vi "Calculate Load Current Array.vi"(8 "error in":errorcluster, 11 "measurement configuration":T1={"Mode of operation"=enum."Perform measurement", "DUT setup time"=1.0, "Source delay"=0.005, "Aperture time"=0.005, "Nominal output voltage"=3.3, "Source pin name"="", "Source sense"=1009, "Source current limit"=25.0, "Source maximum power"=300.0, "Source start voltage"=5.0, "Source stop voltage"=20.0, "Source voltage sweep points"=10, "Use Source voltage array"=FALSE, "Source voltage array"=[], "Load pin name"="", "Load sense"=1009, "Load voltage limit range"=6.0, "Load sweep type"="Logarithmic", "Load start current"=0.1, "Load stop current"=24.0, "Load current sweep points/points per decade"=10, "Use Load current array"=FALSE, "Load current array"=[], "Pin Names for Scope"=[], "vertical range"=[], "vertical offset"=[], "probe attenuation"=[], "vertical coupling"=[], "channel enabled"=[], "input impedance"=[], "max input frequency"=[], "min sample rate"=[], "reference position"=[], "min record length"=[], "enforce realtime"=[]} {"input impedance" items=["1 mega ohm"=0, "50 ohms"=2]; "vertical coupling" items=["AC", "DC", "Ground"]; "Load sense" items=["Local"=1008, "Remote"=1009]; "Source sense" items=["Local"=1008, "Remote"=1009]}) -> (0 "error out":errorcluster, 2 "Load current array size":i32, 3 "Load current array":dbl[](array[numeric]))   [LabVIEW 2021, in "Efficiency And Load Regulation with Pin Map.lvlib"]
uses:
  Efficiency And Load Regulation with Pin Map.lvlib
  Measurement Configuration.ctl
  <instrlib>/niScope/Controls/niScope vertical coupling.ctl
  common/PMIC Common.lvlib
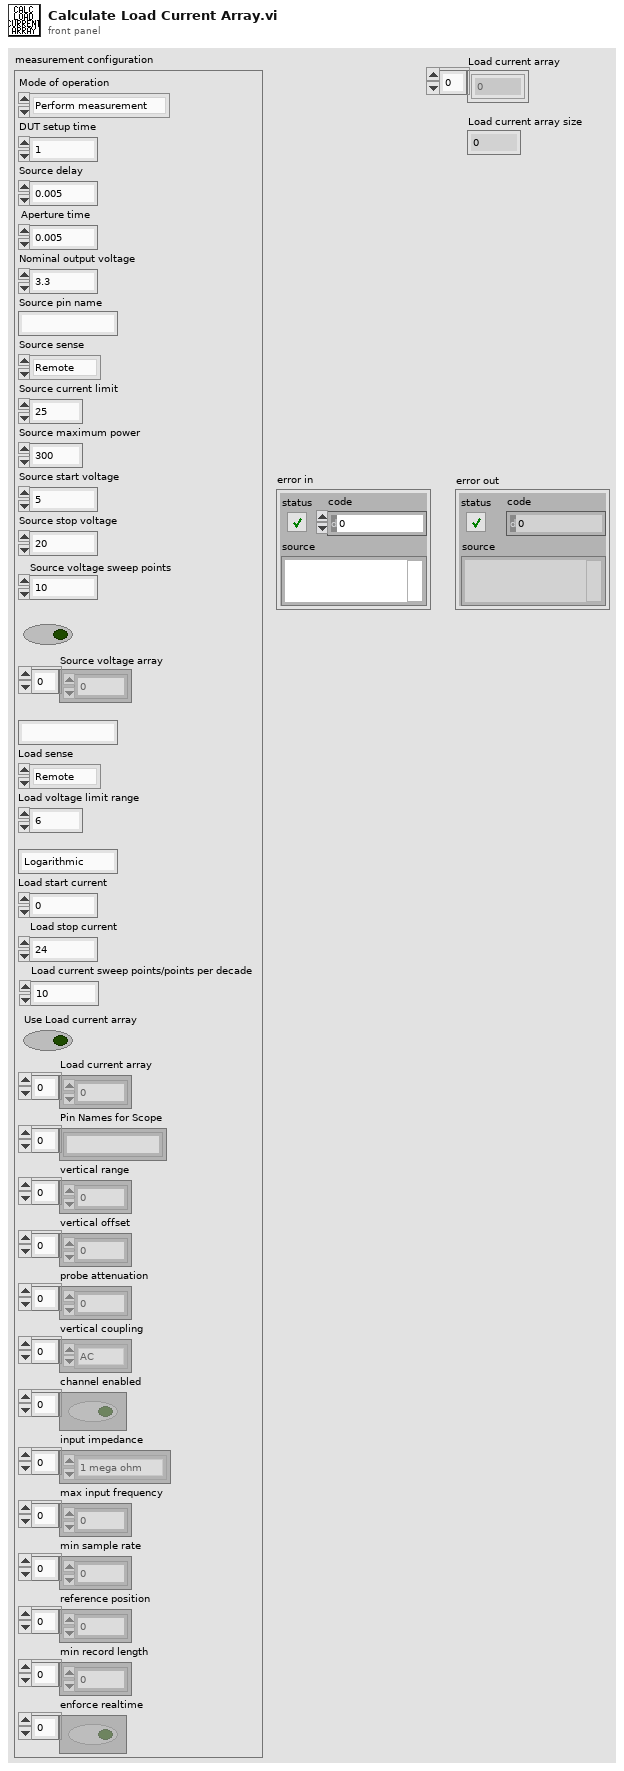
[diagram p1: front panel]
types:
  T1 = typedef "Efficiency And Load Regulation with Pin Map.lvlib/Measurement Configuration.ctl" = cluster{"Mode of operation":enum32{"Power on the DUT", "Perform measurement", "Power off the DUT"}, "DUT setup time":dbl, "Source delay":dbl, "Aperture time":dbl, "Nominal output voltage":dbl, "Source pin name":string, "Source sense":i32, "Source current limit":dbl, "Source maximum power":dbl, "Source start voltage":dbl, "Source stop voltage":dbl, "Source voltage sweep points":i32, "Use Source voltage array":bool, "Source voltage array":dbl[], "Load pin name":string, "Load sense":i32, "Load voltage limit range":dbl, "Load sweep type":string, "Load start current":dbl, "Load stop current":dbl, "Load current sweep points/points per decade":i32, "Use Load current array":bool, "Load current array":dbl[], "Pin Names for Scope":string[], "vertical range":dbl[], "vertical offset":dbl[], "probe attenuation":dbl[], "vertical coupling":T2[], "channel enabled":bool[], "input impedance":u32[], "max input frequency":dbl[], "min sample rate":dbl[], "reference position":dbl[], "min record length":i32[], "enforce realtime":bool[]}
  T2 = typedef "niScope vertical coupling.ctl" = i32
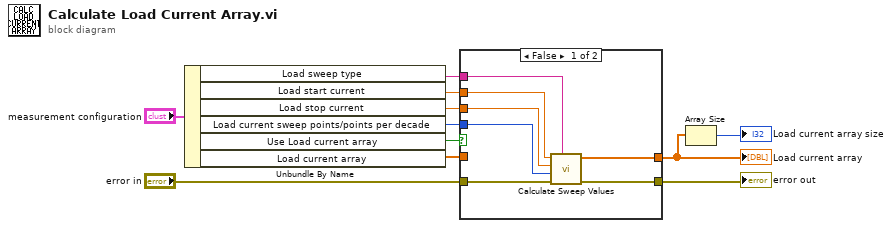
[diagram p0: block diagram]
diagram:
  n1 = Unbundle By Name("measurement configuration") -> ("Load sweep type"=w3:string, "Load start current"=w6:dbl, "Load stop current"=w7:dbl, "Load current sweep points/points per decade"=w8:i32, "Use Load current array"=w10:bool, "Load current array"=w9:dbl[])
  n2 = case shown="False" w10 {
    tunnel: w9 -> [_ w20]
    tunnel: w8 -> [w13 _]
    tunnel: w7 -> [w14 _]
    tunnel: w6 -> [w15 _]
    tunnel: [w12 w20] -> w2
    tunnel: "error in" -> [w18 w19]
    tunnel: [w17 w19] -> w4
    tunnel: w3 -> [w16 _]
    frame False {
      n3 = call "Calculate Sweep Values.vi"("Sweep type"=w16, "error in"=w18, "Points"=w13, "Stop level"=w14, "Start level"=w15) -> ("error out"=w17:errorcluster, "Sweep values"=w12:dbl[])  [unwired: 4 in, 1 out]
    }
    frame True {
    }
  }
  "error out" <- w4
  "Load current array" <- w2
  n4 = Array Size(array=w2) -> (size(s)=→"Load current array size":i32)
